vi "GDSLvIcon_CreateIconPicture.vi"(1 "FrameColor":u32(colorbox), 2 "FrameThickness(1)":u32=1, 3 "HeaderIconIn":u8[][](array[numeric]) format="%x", 4 "BodyIconIn":u8[][](array[numeric]) format="%x", 5 "error in (no error)":errorcluster, 6 "ImageRows(32)":i32=32, 7 "BigSizeIcon(x6)":i32=6, 8 "RowStart(0)":i32, 9 "BgIcon":T1 {"ColorsOkayforiconToBeOnTopOf" format="%x"}) -> (13 "BodyIconOut":u8[][](array[numeric]) format="%x", 15 "WholeIconOut":u8[][](array[numeric]) format="%x", 16 "IconPictureOut":picture, 17 "LargeIconPictureOut(x6)":picture, 18 "BodyOffset":cluster{"X":i32, "Y":i32}, 19 "error out":errorcluster)   [LabVIEW 2014]
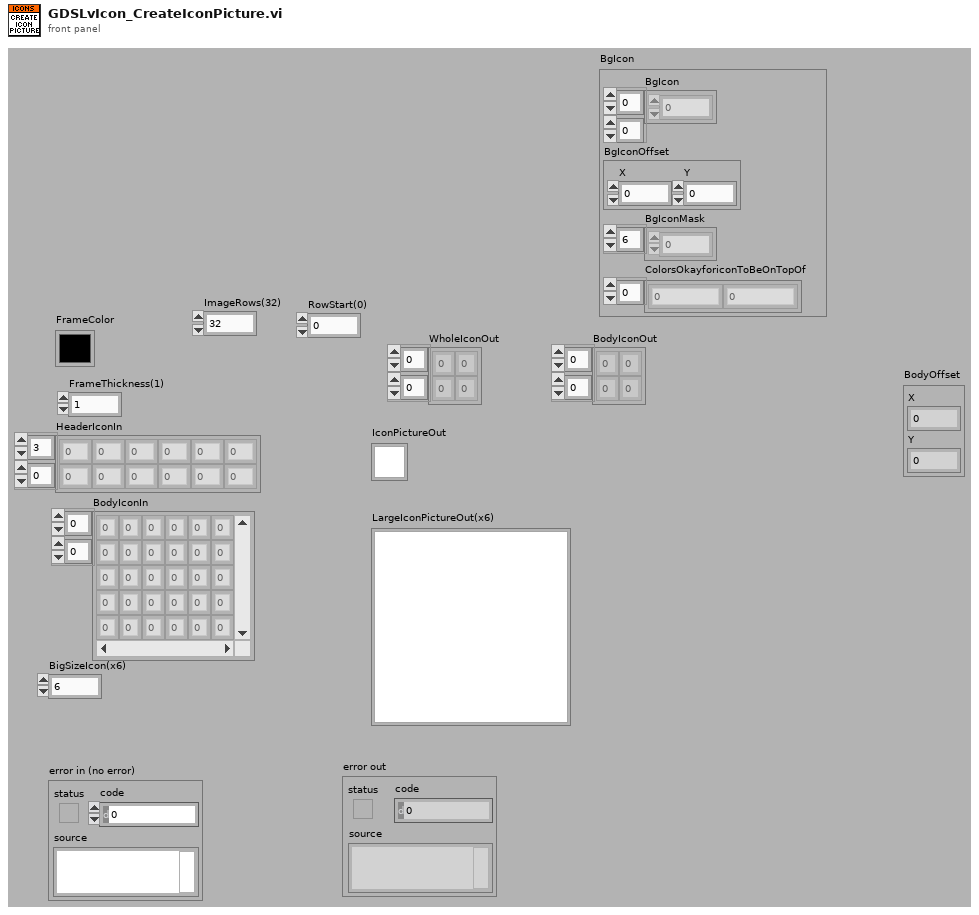
[diagram p1: front panel]
types:
  T1 = cluster{"BgIcon":u8[][], "BgIconOffset":cluster{"X":i32, "Y":i32}, "BgIconMask":u8[], "ColorsOkayforiconToBeOnTopOf":u8[]}
  T2 = cluster{"left":i16, "top":i16, "right":i16, "bottom":i16}
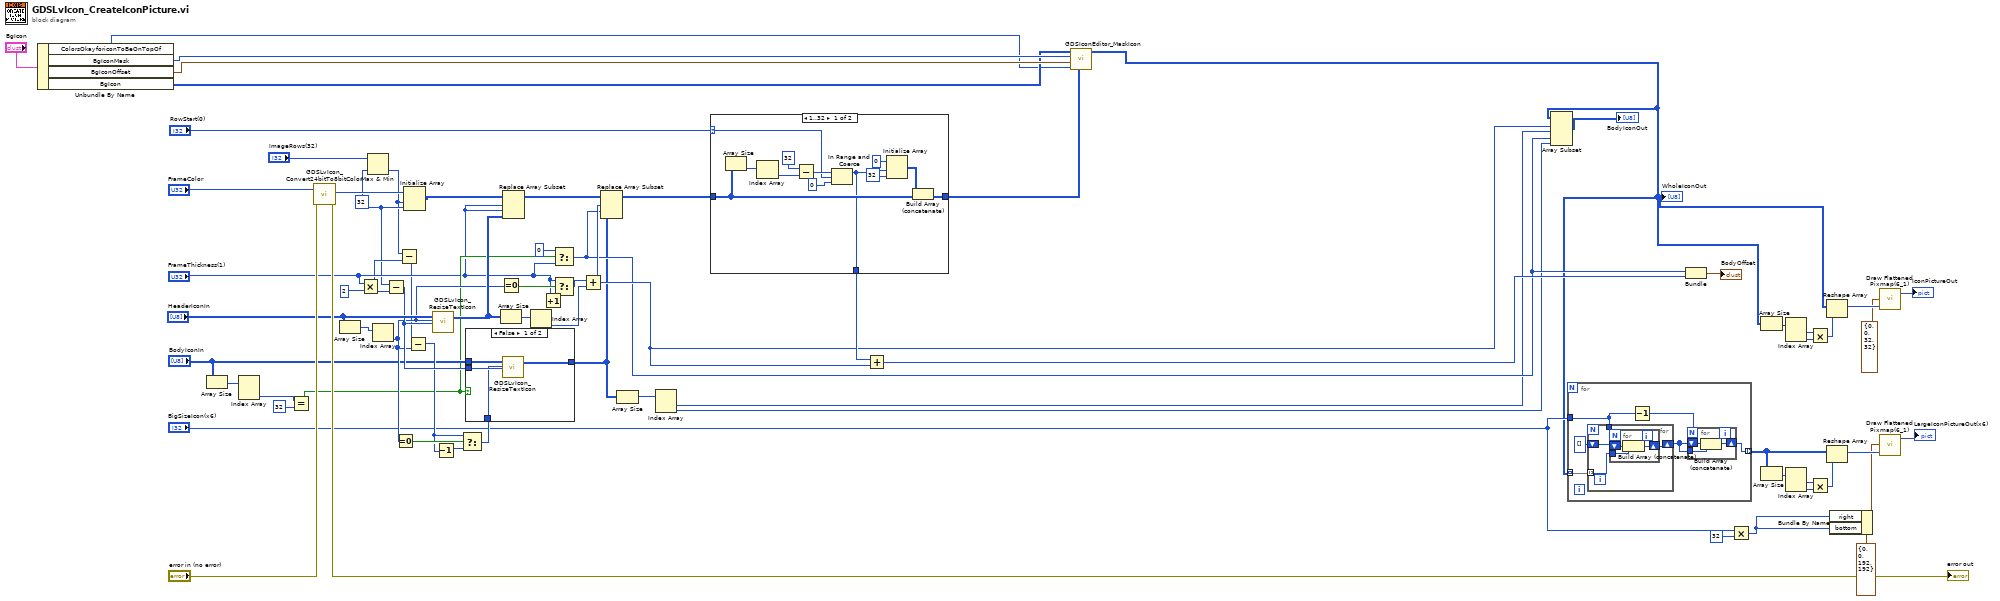
[diagram p0: block diagram]
diagram:
  w13 = 32 ("dimension size")
  n1 = Unbundle By Name("BgIcon") -> ("ColorsOkayforiconToBeOnTopOf"=w1:u8[], "BgIconMask"=w4:u8[], "BgIconOffset"=w19:cluster{"X":i32, "Y":i32}, "BgIcon"=w2:u8[][])
  n2 = Array Size(array="BodyIconIn") -> (size(s)=w31:i32[])
  n3 = Index Array(array=w31) -> (element #2=w18:i32)  [unwired: 2 in, 1 out]
  n4 = Equal?(x=w18, y=32) -> (x = y?=w28:bool)
  n5 = call <resource>:"GDSLvIcon_Convert24bitTo8bitColor.vi"("Color 24bit In"="FrameColor", "error in (no error)"="error in (no error)") -> ("Color out(256)"=w69:u8, "error out"=→"error out":errorcluster)  [unwired: 14 in, 2 out]
  n6 = Array Size(array="HeaderIconIn") -> (size(s)=w46:i32[])
  n7 = Multiply(x="FrameThickness(1)", y=u32 2) -> (x*y=w25:u32)
  n8 = Max & Min(x="ImageRows(32)", y=w13) -> (min(x,y)=w12:i32)  [unwired: 1 out]
  n9 = Index Array(array=w46) -> (element=w34:i32)  [unwired: 1 in]
  n10 = Subtract(x=w13, y=w25) -> (x-y=w45:u32)
  n11 = Equal To 0?(x=w34) -> (x = 0?=w40:bool)
  n12 = Subtract(x=w12, y=w25) -> (x-y=w24:u32)
  n13 = Initialize Array(w69, w12, w13) -> (w68:u8[][])
  n14 = Subtract(x=w24, y=w34) -> (x-y=w38:u32)
  n15 = call <resource>:"GDSLvIcon_ResizeTextIcon.vi"("IconIn"="HeaderIconIn", "Rows/Height"=w34, "Columns/Width"=w45) -> ("IconOut"=w49:u8[][])  [unwired: 15 in, 1 out]
  n16 = Decrement(x=w38) -> (x-1=w39:u32)
  n17 = Select(t=w38, s=w40, f=w39) -> (s? t:f=w37:u32)
  n18 = case shown="False" w28 {
    tunnel: [w75 w76] -> w9
    tunnel: w45 -> [w74 _]
    tunnel: w37 -> [w73 _]
    tunnel: "BodyIconIn" -> [w72 w76]
    frame False {
      n19 = call <resource>:"GDSLvIcon_ResizeTextIcon.vi"("IconIn"=w72, "Rows/Height"=w73, "Columns/Width"=w74) -> ("IconOut"=w75:u8[][])  [unwired: 15 in, 1 out]
    }
    frame True {
    }
  }
  n20 = Equal To 0?(x=w34) -> (x = 0?=w36:bool)
  n21 = Array Size(array=w49) -> (size(s)=w66:i32[])
  n22 = Replace Array Subset(array=w68, new element=w49, index (row)="FrameThickness(1)", index (col)="FrameThickness(1)") -> (w67:u8[][])
  n23 = Index Array(array=w66) -> (element=w58:i32)  [unwired: 1 in]
  n24 = Increment(x="FrameThickness(1)") -> (x+1=w35:u32)
  n25 = Select(t=u32 0, s=w28, f="FrameThickness(1)") -> (s? t:f=w10:u32)
  n26 = Select(t="FrameThickness(1)", s=w36, f=w35) -> (s? t:f=w33:u32)
  n27 = Add(x=w33, y=w58) -> (x+y=w11:u32)
  n28 = Replace Array Subset(array=w67, new element=w9, index (row)=w11, index (col)=w10) -> (w22:u8[][])
  n29 = Array Size(array=w9) -> (size(s)=w8:i32[])
  n30 = Index Array(array=w8) -> (element #1=w7:i32, element #2=w6:i32)  [unwired: 2 in]
  n31 = case shown="1..32" "RowStart(0)" {
    selector: "RowStart(0)" -> [w78 _]
    tunnel: [w85 w89] -> w21
    tunnel: w22 -> [w84 w89]
    tunnel: [w77 _] -> w17
    frame 1..32 {
      n32 = Array Size(array=w84) -> (size(s)=w83:i32[])
      n33 = Index Array(array=w83) -> (element=w81:i32)  [unwired: 1 in]
      n34 = Subtract(x=32 ("dimension size"), y=w81) -> (x-y=w79:i32)
      n35 = In Range and Coerce(upper limit=w79, x=w78, lower limit=0) -> (coerced(x)=w77:i32)  [unwired: 1 out]
      n36 = Initialize Array(u8 0 ("element"), w77, 32 ("dimension size")) -> (w86:u8[][])
      n37 = Build Array (concatenate)(w86, w84) -> (w85:u8[][])
    }
    frame Default {
    }
  }
  n38 = Add(x=w17, y=w11) -> (x+y=w15:u32)
  n39 = call <resource>:"GDSIconEditor_MaskIcon.vi"("BgIcon"=w21, "ColorsOkayforiconToBeOnTopOf"=w1, "BgIconOffset"=w19, "BgIconMask"=w4, "IconIn"=w2) -> ("IconOut"=w3:u8[][])  [unwired: 6 in]
  "WholeIconOut" <- w3
  n40 = Array Subset(array=w3, index (row)=w11, length (row)=w7, index (col)=w10, length (col)=w6) -> (→"BodyIconOut":u8[][])
  n41 = for {
    tunnel: w3 -> [w95] mode=indexing
    tunnel: [w93] -> w60 mode=indexing
    tunnel: "BigSizeIcon(x6)" -> [w90]
    n42 = for {
      tunnel: w95 -> [w102] mode=indexing
      shift-right: [w100] -> w92
      shift-left: u8[] [] -> [w101]
      tunnel: w90 -> [w99]
      n43 = for {
        N: w99 -> [_]
        tunnel: w102 -> [w105]
        shift-right: [w103] -> w100
        shift-left: w101 -> [w104]
        n44 = Build Array (concatenate)(w104, w105) -> (w103:u8[])
      }
    }
    n45 = Decrement(x=w90) -> (x-1=w91:i32)
    n46 = for {
      N: w91 -> [_]
      tunnel: w92 -> [w98]
      shift-right: [w96] -> w93
      shift-left: w92 -> [w97]
      n47 = Build Array (concatenate)(w97, w98) -> (w96:u8[])
    }
  }
  n48 = Bundle("FrameThickness(1)"=w10, w15) -> (→"BodyOffset":cluster{"FrameThickness(1)":u32, u32})  [unwired: 1 in]
  n49 = Multiply(x="BigSizeIcon(x6)", y=32) -> (x*y=w41:i32)
  n50 = Array Size(array=w3) -> (size(s)=w52:i32[])
  n51 = Array Size(array=w60) -> (size(s)=w64:i32[])
  n52 = Index Array(array=w52) -> (element #1=w54:i32, element #2=w53:i32)  [unwired: 2 in]
  n53 = Index Array(array=w64) -> (element #1=w62:i32, element #2=w63:i32)  [unwired: 2 in]
  n54 = Multiply(x=w54, y=w53) -> (x*y=w55:i32)
  n55 = Multiply(x=w62, y=w63) -> (x*y=w61:i32)
  n56 = Reshape Array(w3, w55) -> (w56:u8[])
  n57 = Reshape Array(w60, w61) -> (w59:u8[])
  n58 = Bundle By Name(cluster=T2 {"left"=0, "top"=0, "right"=192, "bottom"=192} ("rect"), "right"=w41, "bottom"=w41) -> (w43:T2)
  n59 = call <vilib>:"Draw Flattened Pixmap(6_1).vi"("rect"=T2 {"left"=0, "top"=0, "right"=32, "bottom"=32}, "flattened pixmap data"=w56) -> ("new picture"=→"IconPictureOut":picture)  [unwired: 7 in]
  n60 = call <vilib>:"Draw Flattened Pixmap(6_1).vi"("rect"=w43, "flattened pixmap data"=w59) -> ("new picture"=→"LargeIconPictureOut(x6)":picture)  [unwired: 7 in]
